vi "CC Read Channels from TDMS File.vi"(8 "error in (no error)":errorcluster, 10 "Sources":string[](array[string]), 11 "ItemNames":string[](array[string])) -> (0 "error out":errorcluster, 1 "units":string[](array[string]), 2 "Y Axes":i32[](array[numeric]), 3 "XY Graph":cluster{timestamp[], dbl[]}[](graph))   [LabVIEW 2024]
uses:
  CC enum Current Values Action.ctl
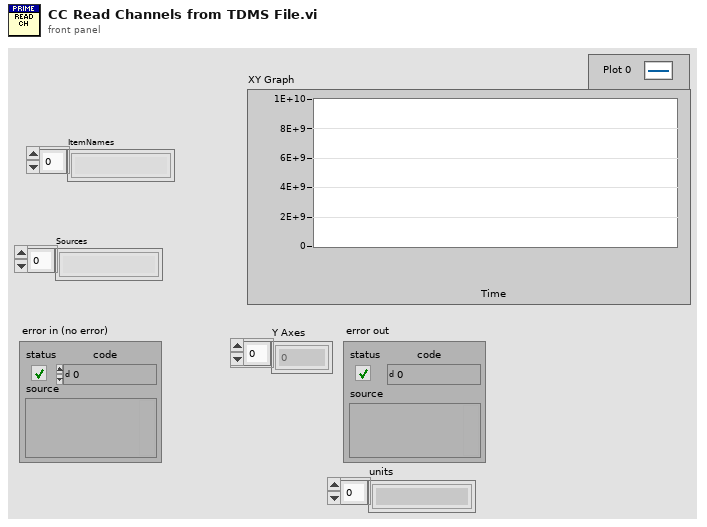
[diagram p1: front panel]
types:
  T1 = typedef "CC enum Current Values Action.ctl" = enum16{"Init", "Write Item", "Write Array", "Read Item", "Read Array", "Read All", "Add Channels", "New File", "Add Message", "Get Current Values", "Close"}
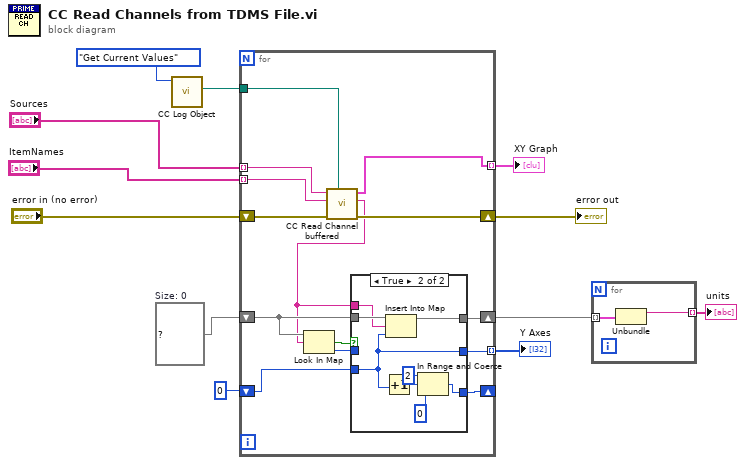
[diagram p0: block diagram]
diagram:
  w9 = map{string, i32} {}  # Size: 0
  n1 = call "CC Log Object.vi"("Action"=CC_enum_Current_Values_Action."Get Current Values") -> ("Current File"=w1:path)  [unwired: 8 in, 2 out]
  n2 = for {
    tunnel: [w19] -> w12 mode=indexing
    shift-right: [w15] -> w3
    shift-left: "error in (no error)" -> [w16]
    tunnel: "Sources" -> [w18] mode=indexing
    tunnel: "ItemNames" -> [w17] mode=indexing
    shift-right: [w22] -> w7
    shift-left: w9 -> [w23]
    shift-right: [w21] -> _
    shift-left: 0 -> [w24]
    tunnel: [w20] -> w5 mode=indexing
    tunnel: w1 -> [w13]
    n3 = call "CC Read Channel buffered.vi"("Current File"=w13, "error in (no error)"=w16, "channel"=w17, "group"=w18) -> ("error out"=w15:errorcluster, "Units"=w14:string, "Data"=w19:cluster{"timestamps":timestamp[], "data":dbl[]})  [unwired: 5 in]
    n4 = Look In Map(map=w23, key=w14) -> (key not found?=w26:bool, value=w25:i32)  [unwired: 1 in]
    n5 = case shown="True" w26 {
      tunnel: w25 -> [w27 _]
      tunnel: w24 -> [w28 w30]
      tunnel: w23 -> [w29 w37]
      tunnel: [w29 w36] -> w22
      tunnel: w14 -> [_ w35]
      tunnel: [w28 w31] -> w21
      tunnel: [w27 w30] -> w20
      frame False {
      }
      frame True {
        n6 = Increment(x=w30) -> (x+1=w34:i32)
        n7 = Insert Into Map(map in=w37, key=w35, value=w30) -> (map out=w36:map{string, i32})  [unwired: 2 out]
        n8 = In Range and Coerce(upper limit=2, x=w34, lower limit=0) -> (coerced(x)=w31:i32)  [unwired: 1 out]
      }
    }
  }
  "error out" <- w3
  "XY Graph" <- w12
  "Y Axes" <- w5
  n9 = for {
    tunnel: w7 -> [w39] mode=indexing
    tunnel: [w38] -> w6 mode=indexing
    n10 = Unbundle(w39) -> (w38:string)  [unwired: 1 out]
  }
  "units" <- w6
